vi "tablice2.vi"() -> ()   [LabVIEW 2019]
panel:
  out "Rozmiar tablicy":i32[](array[numeric])
  out "Index min":i32[](array[numeric])
  out "Index max":i32[](array[numeric])
  out "Tablica wyjsciowa":dbl[][](array[numeric])
  out "Suma":dbl
  out "Wartosc min":dbl
  out "Wartosc max":dbl
  in  "Indeks kolumny":dbl
  in  "Index wiersza":dbl
  in  "Wypłenienie tablicy wstawianej":dbl
  out "Tablica wstawiana":dbl[][](array[numeric])
  in  "Wprowadzanie danych":dbl[][](array[numeric])
  in  "?":bool
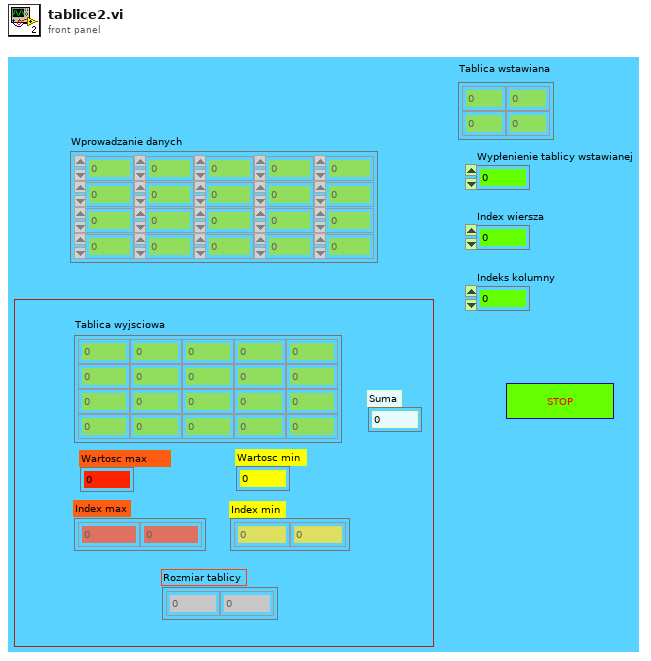
[diagram p1: front panel]
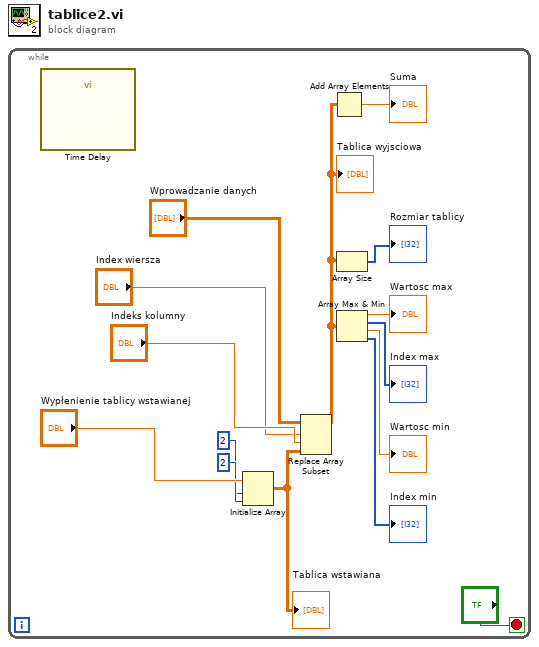
[diagram p0: block diagram]
diagram:
  n1 = while {
    stop <- "?" stop-if-true
    n2 = call "Time Delay"() -> ()  [unwired: 11 in, 1 out]
    n3 = Initialize Array("Wypłenienie tablicy wstawianej", 2 ("dimension size"), 2 ("dimension size")) -> (w1:dbl[][])
    "Tablica wstawiana" <- w1
    n4 = Replace Array Subset(array="Wprowadzanie danych", new element=w1, index (row)="Index wiersza", index (col)="Indeks kolumny") -> (w4:dbl[][])
    "Tablica wyjsciowa" <- w4
    n5 = Add Array Elements(numeric array=w4) -> (sum=→"Suma":dbl)
    n6 = Array Size(array=w4) -> (size(s)=→"Rozmiar tablicy":i32[])
    n7 = Array Max & Min(array=w4) -> (max value=→"Wartosc max":dbl, max index (indices)=→"Index max":i32[], min value=→"Wartosc min":dbl, min index (indices)=→"Index min":i32[])
  }
